vi "Load Mouse LLB.vi"(8 "error in (no error)":errorcluster, 11 "Mouse LLB":path) -> (0 "error out":errorcluster, 2 "Name":string, 3 "Mouse":refnum<class "Mouse.lvclass">)   [LabVIEW 2020]
uses:
  Mouse/Mouse.lvclass
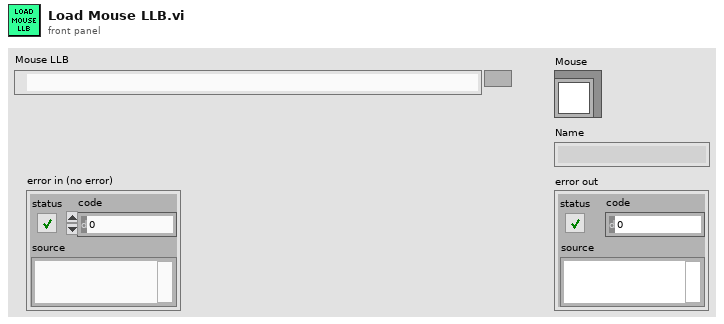
[diagram p1: front panel]
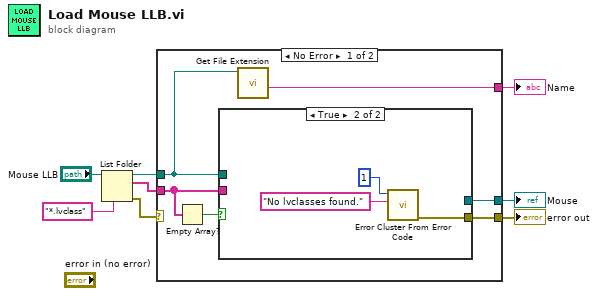
[diagram p0: block diagram]
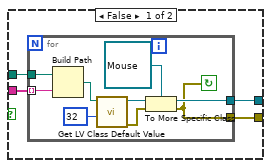
[diagram p2: hidden frame]
diagram:
  n1 = List Folder(path="Mouse LLB", pattern="*.lvclass") -> (path out=w5:path, filenames=w6:string[], error out=w4:errorcluster)  [unwired: 2 in, 1 out]
  n2 = case shown="No Error" w4 {
    selector: w4 -> [_ w31]
    tunnel: [w14 _] -> w2
    tunnel: [w13 w31] -> w3
    tunnel: w6 -> [w10 _]
    tunnel: w5 -> [w12 _]
    tunnel: [w11 _] -> w1
    frame No Error {
      n3 = Empty Array?(array=w10) -> (empty?=w9:bool)
      n4 = case shown="True" w9 {
        tunnel: [w18 _] -> w14
        tunnel: [w17 w28] -> w13
        tunnel: w12 -> [w16 _]
        tunnel: w10 -> [w15 _]
        frame False {
          n5 = for {
            tunnel: [w26] -> w18
            tunnel: [w24] -> w17
            tunnel: w16 -> [w23]
            tunnel: w15 -> [w22] mode=indexing
            stop <- w24 continue-if-true
            n6 = Build Path(base path=w23, name or relative path=w22) -> (appended path=w19:path)
            n7 = call <vilib>:"Get LV Class Default Value.vi"("options"=u32 32, "class path"=w19) -> ("error out"=w20:errorcluster, "object"=w21:refnum<class>)  [unwired: 8 in]
            n8 = To More Specific Class(target class=refnum<class "Mouse.lvclass"> refnum ("Maze.lvlib:Mouse.lvclass"), reference=w21, error in=w20) -> (specific class reference=w26:refnum<class "Mouse.lvclass">, error out=w24:errorcluster)
          }
        }
        frame True {
          n9 = call <vilib>:"Error Cluster From Error Code.vi"("error message (\"\")"="No lvclasses found." ("error message (\"\")"), "error code (0)"=1) -> ("error out"=w28:errorcluster)  [unwired: 7 in]
        }
      }
      n10 = call <vilib>:"Get File Extension.vi"("file"=w12) -> ("filename without extension"=w11:string)  [unwired: 6 in, 4 out]
    }
    frame Error {
    }
  }
  "error out" <- w3
  "Mouse" <- w2
  "Name" <- w1
